vi "Write to Host Bound FIFO (U256).vi"(7 "Host FIFO":refnum<k21>="To Host", 8 "Input Valid":bool, 11 "Input Data":T1) -> (2 "Data Written":bool, 3 "data out":u64, 6 "Ready For Input":bool)   [LabVIEW 2012]
doc: "<b> This VI transfers U256 data to Host in U64 Chunks </b>\n\nIt takes 4 Ticks for this VI to insert data into Host FIFO if there is space available in the Host FIFO. The VI will retry sending data into Host FIFO until space is available. Further it will send \"Ready for Input\" signal to upstream block as when it can accept data."
uses:
  <vilib>/rvi/DataTransferAndStorage/Container/Common/niFpgaContainerMetaDataKey.ctl
  <vilib>/rvi/DataTransferAndStorage/Container/Common/niFpgaContainerState.ctl
  <vilib>/rvi/DataTransferAndStorage/Container/Common/niFpgaDataTypeControl.ctl
  <vilib>/rvi/DataTransferAndStorage/Container/Common/niFpgaContainerImplementationControl.ctl
  <vilib>/rvi/DataTransferAndStorage/Container/Common/niFpgaContainerArbitrationOptionsControl.ctl
  <vilib>/rvi/DataTransferAndStorage/Container/Common/niFpgaTransferTypeControl.ctl
  <vilib>/rvi/DataTransferAndStorage/Container/Common/niFpgaContainerInitializationParameters.ctl
  <vilib>/rvi/Memory/Memory_Types/niFpgaMemoryInterfaceConfiguration.ctl
  <vilib>/rvi/FIFO/Fifo_Types/niFpgaFifoControlLogicControl.ctl
  <vilib>/rvi/DataTransferAndStorage/Container/Common/niFpgaContainerGetUniqueNameForEmu.vi
  <vilib>/rvi/DataTransferAndStorage/Container/Common/niFpgaContainerSetEmuInfo.vi
  <vilib>/rvi/eio/common/nirviEmuReportErrorAndStop.vi
  <vilib>/rvi/DataTransferAndStorage/Container/Common/niFpgaContainerExecOnDevCompGetState.vi
  <vilib>/rvi/FIFO/Fifo_Resource/nirvififoEmulationSetSize.vi
  <vilib>/rvi/interface/RandomDataEmulation/nirviRandomDataFPGAFIFO.vi
  <vilib>/rvi/interface/RandomDataEmulation/niFpgaRandomDataHandleErrors.vi
  <vilib>/rvi/Emulation/niFpgaSctlEmulationGetInTimedLoop.vi
  <vilib>/rvi/Emulation/niFpgaSctlEmulationFifoFullMgr.vi
  <vilib>/rvi/errors/niFpgaSetErrorForExecOnDevCompSimple.vi
  <vilib>/rvi/interface/RandomDataEmulation/nirviRandomDataAcquireLock.vi
  <vilib>/rvi/interface/RandomDataEmulation/nirviRandomDataCheckExitLoopConditions.vi
  <vilib>/rvi/interface/RandomDataEmulation/nirviRandomDataReleaseLock.vi
  <vilib>/rvi/interface/RandomDataEmulation/nirviFPGAContextMergeError.vi
  <vilib>/rvi/Emulation/niFpgaSctlEmulationResourceMgr.vi
  <vilib>/rvi/LocalResourceManager/LocalResourceManager.xnode
  <vilib>/rvi/DataTransferAndStorage/Container/XNode/niFpgaContainer.xnode
  <vilib>/rvi/FIFO/Fifo_Resource/niFpgaFifoEmulationRefIn.vi
  <vilib>/rvi/FIFO/Fifo_Resource/niFpgaFifoEmulationRefInMultiElement.vi
  <instrlib>/FlexRIO/Libraries/Helper VIs/NI FlexRIO Helper VIs.lvlib
panel:
  out "data valids written":u64
  out "data validsafter handshanke":u64
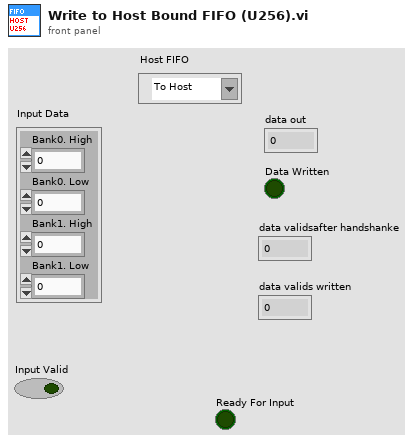
[diagram p1: front panel]
types:
  T1 = cluster{"Bank0. High":u64, "Bank0. Low":u64, "Bank1. High":u64, "Bank1. Low":u64}
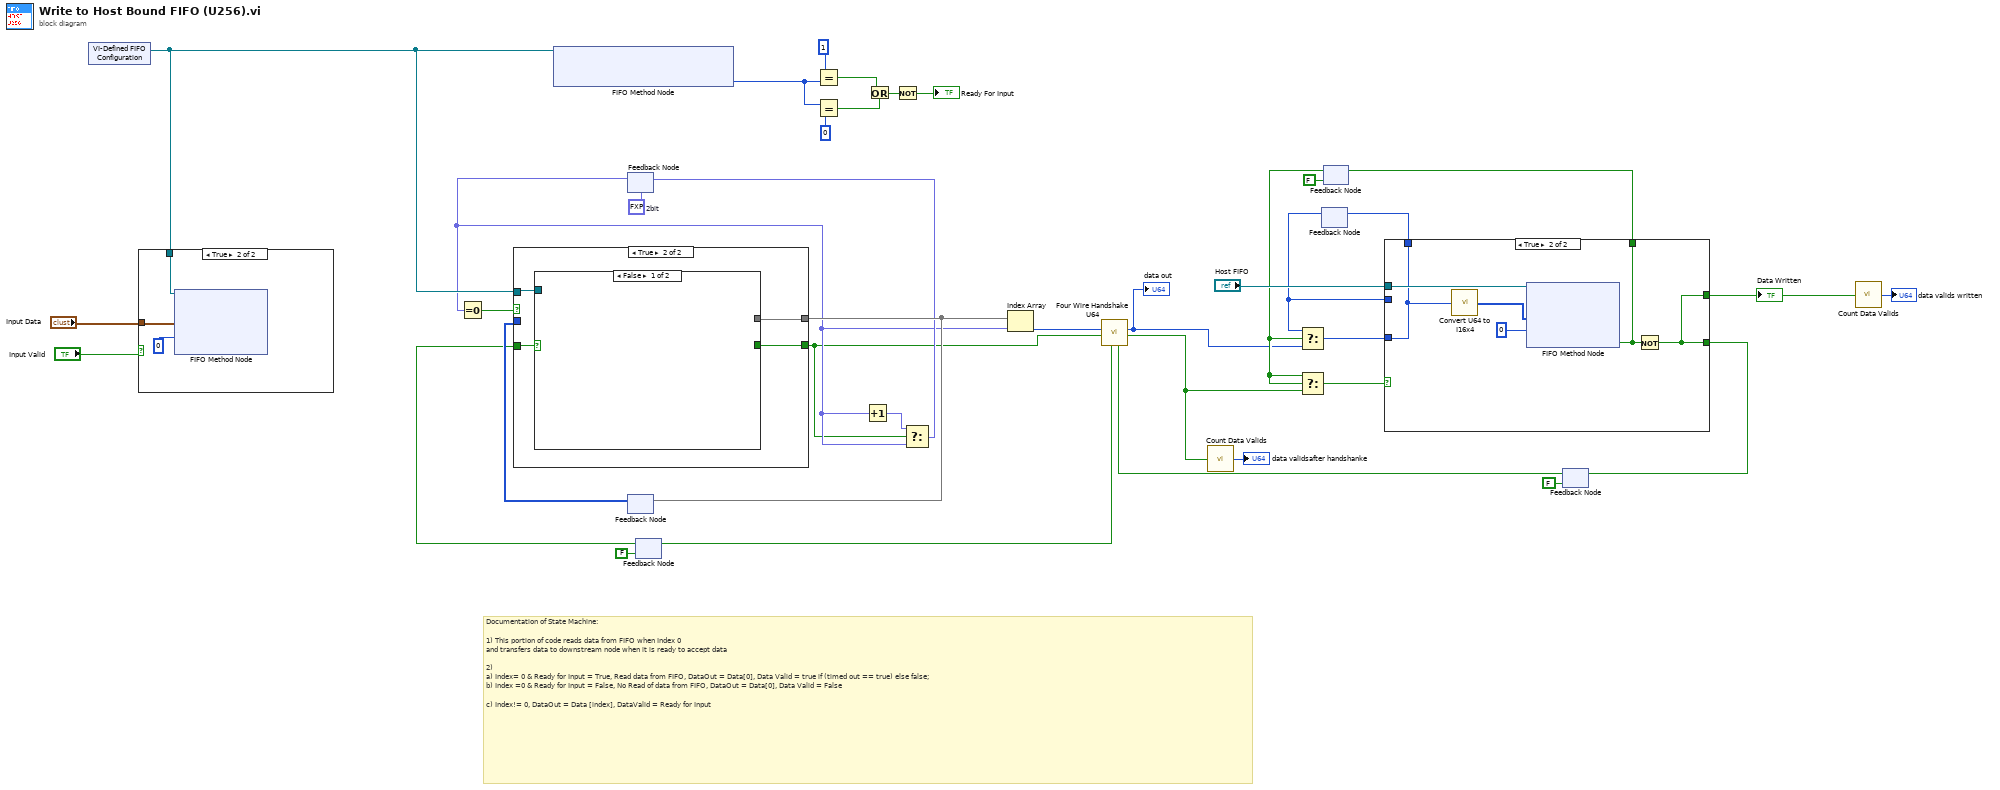
[diagram p0: block diagram]
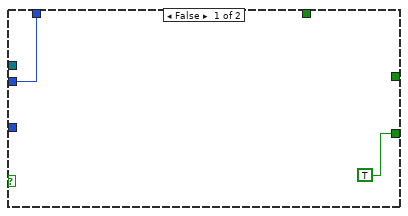
[diagram p2: hidden frame]
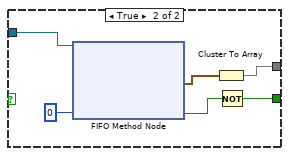
[diagram p4: hidden frame]
diagram:
  w26 = fxp<+,2,2> 0.0  # 2bit
  # "Documentation of State Machine:\n\n1) This portion of code reads data from FIFO when Index 0\nand transfers data to downstream node when it is ready to accept data\n\n2) \na) Index= 0 & Ready for Input = True, Read data from FIFO, DataOut = Data[0], Data Valid = true if (timed out == true) else false; \nb) Index =0 & Ready for Input = False, No Read of data from FIFO, DataOut = Data[0], Data Valid = False\n\nc) Index!= 0, DataOut = Data [index], DataValid = Ready for Input"
  n1 = xnode "VI-Defined FIFO Configuration"() -> ("FIFO Out"=w31:refnum<k21>)
  n2 = case shown="True" "Input Valid" {
    tunnel: w31 -> [_ w41]
    tunnel: "Input Data" -> [_ w40]
    frame False {
    }
    frame True {
      n3 = xnode ("FIFO Method Node")("Element"=w40, "Timeout"=0, "FIFO In"=w41) -> ()  [unwired: 2 out]
    }
  }
  n4 = xnode ("FIFO Method Node")("FIFO In"=w31) -> ("Number of Elements to Write"=w34:u32)  [unwired: 1 out]
  n5 = feedback #1(w26) -> (w20:fxp<+,2,2>)
  n6 = Equal To 0?(x=w20) -> (x = 0?=w24:bool)
  n7 = feedback #2() -> (w28:u64[])  [unwired: 1 in]
  n8 = feedback #3(FALSE ("ready for input")) -> (w23:bool)
  n9 = case shown="True" w24 {
    tunnel: [w42 w45] -> w17
    tunnel: w31 -> [_ w47]
    tunnel: [w43 w46] -> w27
    tunnel: w28 -> [w43 _]
    tunnel: w23 -> [w42 w44]
    frame False {
    }
    frame True {
      n10 = case shown="False" w44 {
        tunnel: w47 -> [_ w53]
        tunnel: [_ w49] -> w46
        tunnel: [_ w48] -> w45
        frame False {
        }
        frame True {
          n11 = xnode ("FIFO Method Node")("Timeout"=0, "FIFO In"=w53) -> ("Element"=w50:T1, "Timed Out?"=w52:bool)  [unwired: 1 out]
          n12 = Cluster To Array(cluster=w50) -> (array=w49:u64[])
          n13 = Not(x=w52) -> (.not. x?=w48:bool)
        }
      }
    }
  }
  n14 = feedback-in #2(w27) -> ()
  n15 = Equal?(x=u32 1 ("y"), y=w34) -> (x = y?=w36:bool)
  n16 = Equal?(x=w34, y=u32 0) -> (x = y?=w35:bool)
  n17 = Increment(x=w20) -> (x+1=w22:fxp<+,2,2>)
  n18 = Or(x=w36, y=w35) -> (x .or. y?=w38:bool)
  n19 = Not(x=w38) -> (.not. x?=→"Ready For Input":bool)
  n20 = Select(t=w22, s=w17, f=w20) -> (s? t:f=w21:fxp<+,2,2>)
  n21 = feedback-in #1(w21) -> ()
  n22 = Index Array(array=w27, index=w20) -> (element=w18:u64)
  n23 = feedback #4() -> (w1:u64)  [unwired: 1 in]
  n24 = feedback #5(FALSE ("Timed Out?")) -> (w6:bool)
  n25 = feedback #6(FALSE) -> (w13:bool)
  n26 = call <instrlib>:"Four Wire Handshake U64.vi"("ready for output"=w13, "data valid"=w17, "Data"=w18) -> ("valid out"=w5:bool, "data out"=w2:u64, "ready for input"=w15:bool)  [unwired: 5 in, 1 out]
  "data out" <- w2
  n27 = feedback-in #3(w15) -> ()
  n28 = call <userlib>:"Count Data Valids.vi"("Data Valid"=w5) -> ("Counter"=→"data validsafter handshanke":u64)  [unwired: 14 in]
  n29 = Select(t=w1, s=w6, f=w2) -> (s? t:f=w8:u64)
  n30 = Select(t=w6, s=w6, f=w5) -> (s? t:f=w4:bool)
  n31 = case shown="True" w4 {
    tunnel: "Host FIFO" -> [_ w61]
    tunnel: [TRUE w59] -> w11
    tunnel: [_ w59] -> w10
    tunnel: [_ w58] -> w9
    tunnel: w8 -> [_ w57]
    tunnel: [w55 w57] -> w7
    tunnel: w1 -> [w55 _]
    frame False {
    }
    frame True {
      n32 = call <userlib>:"Convert U64 to I16x4.vi"("U64"=w57) -> ("4xI16 Array"=w56:i16[])  [unwired: 14 in]
      n33 = xnode ("FIFO Method Node")("Element"=w56, "Timeout"=0, "FIFO In"=w61) -> ("Timed Out?"=w58:bool)  [unwired: 1 out]
      n34 = Not(x=w58) -> (.not. x?=w59:bool)
    }
  }
  "Data Written" <- w10
  n35 = feedback-in #4(w7) -> ()
  n36 = feedback-in #5(w9) -> ()
  n37 = feedback-in #6(w11) -> ()
  n38 = call <userlib>:"Count Data Valids.vi"("Data Valid"=w10) -> ("Counter"=→"data valids written":u64)  [unwired: 14 in]
